vi "COD主界面（列队使用）.vi"() -> (8 "多列列表框":i32(listbox))   [LabVIEW 2016, in "斯坦道CODMn.lvlib"]
uses:
  <vilib>/Utility/miscctls.llb/LVPointTypeDef.ctl
  <vilib>/Plasmionique/MB Master/MB_Master_Serial/MB_Master_Serial.lvclass
  D:/Program Files (x86)/National Instruments/LabVIEW 2016/vi.lib/Plasmionique/MB Master/MB_Master/MB_Master.lvclass
  <vilib>/Plasmionique/MB Master/MB Master.lvlib
  <vilib>/ptbypt/NI_PtbyPt.lvlib
  PLC/PLC.lvlib
panel:
  out "测量数据区":T1 {"单位" items=["ug/L", "mg/L", "ppm", "mg/m3", "cm", "ppb", "ug/m3", "%", "nmol/mol", "umol/mol", "MPN/L", "MPN/100ml", "ng/m3", "NTU", "无量纲", "ms/cm", "us/cm", "℃", "mV", "万个/L"]}
  out "启动选择 3":u16(ring) items=["水样测试", "标样核查", "零点核查", "加标回收", "平行样", "校零", "校标", ""]
  out "加热":bool
  out "搅拌":bool
  out "进硫酸":bool
  out "进草酸钠":bool
  out "进高锰酸钾":bool
  out "进加标回收样":bool
  out "进质控样":bool
  out "进标液":bool
  out "进蒸馏水":bool
  out "进水样":bool
  in  "定时启动":bool
  out "设置值":dbl
  out "系统时间":timestamp
  in  "时间校准":bool
  out "仪器时间":timestamp
  in  "修正系数 2":dbl
  in  "浓度 2":dbl
  in  "温度":dbl
  out "秒":u16
  out "分":u16
  in  "data in":T2
  out "数值":i32
  out "报警簇":T3
  out "读取参数":u16[](array[numeric])
  out "循环次数":i32
  out "DATABASE":u16[](array[numeric])
  out "Registers":u16[](array[numeric])
  in  "枚举":enum16{"读取数据", "写入数据", "读取写入DATABASE", "读取参数"}(ring)
  in  "Slave ID":u8=1
  in  "Serial Config":T4={"baud rate (bps)"=115200, "stop bits"=10, "parity"=0, "flow control"=0, "timeout"=1000, "retries"=1} {"stop bits" items=["1.0"=10, "1.5"=15, "2.0"=20]; "flow control" items=["None", "XON/XOFF", "RTS/CTS", "XON/XOFF & RTS/CTS", "DTR/DSR", "XON/XOFF & DTR/DSR"]; "parity" items=["None", "Odd", "Even", "Mark", "Space"]}
  out "COD浓度（mg/L)":dbl
  out "table 输入":string
  out "columns":string[](array[string])
  in  "保存":bool
  out "data":T5
  in  "温度 2":dbl
  in  "恒温时间":dbl
  in  "浓度":dbl
  in  "修正系数":dbl
  in  "基本量程":enum16{"10mL", "20mL"}(ring)
  in  "水样":dbl
  in  "蒸馏水":dbl
  in  "标液":dbl
  in  "质控样":dbl
  in  "加标回收":dbl
  in  "草酸钠":dbl
  in  "高锰酸钾":dbl
  in  "硫酸":dbl
  in  "关闭":bool
  in  "零点泵计量数 2":dbl
  in  "标度泵计量数 2":dbl
  in  "标样浓度 2":dbl
  out "进样管":dbl
  out "高锰酸钾":dbl
  out "草酸钠":dbl
  out "硫酸":dbl
  out "标度滴定值":dbl
  out "零点滴定值":dbl
  in  "启动":bool
  in  "故障清除":bool
  out "排液故障":bool
  out "进水样超量程":bool
  out "模式（受控）":u16
  out "ORP显示":dbl
  out "温度":dbl
  out "标样核查标记":bool
  out "平行样测量":bool
  out "加标回收测量":bool
  out "质控样测量":bool
  out "待机":bool
  out "校标错误":bool
  out "校零错误":bool
  out "测量错误":bool
  out "草酸钠报警":bool
  out "高锰酸钾报警":bool
  out "加热故障":bool
  out "温控器故障":bool
  out "ORP故障":bool
  out "排液标记":bool
  out "故障标记":bool
  out "校标标记":bool
  out "校零标记":bool
  out "通讯状态":bool
  out "水样测量":bool
  in  "参数配置":bool
  in  "VISA resource name":refnum<visa-resource-name>="COM4" caption="VISA资源名称"
  in  "停止":bool
  in  "单步启动":bool
  # "测量时间："
  # "水样~加标回收"
  # "mV"
  # "℃"
  # "注：遇到加热故障和排液故障时仪器不能正常启动，\n必须排查故障并点击报警清除按钮方可运行。"
  # "基本参数设置"
  # "泵计量参数设置"
  # "校零校标结果"
  # "加热恒温温度（℃）："
  # "水样："
  # "高锰酸钾："
  # "校零结果："
  # "校零滴定值："
  # "恒温时间（分钟）："
  # "蒸馏水："
  # "草酸钠："
  # "校标结果："
  # "标度滴定值："
  # "零点泵计量值："
  # "标准液浓度（mg/L）："
  # "标液："
  # "硫酸："
  # "标样浓度："
  # "标度泵计量值："
  # "修正系数："
  # "质控样："
  # "加标回收样："
  # "基本量程（20mL可选）："
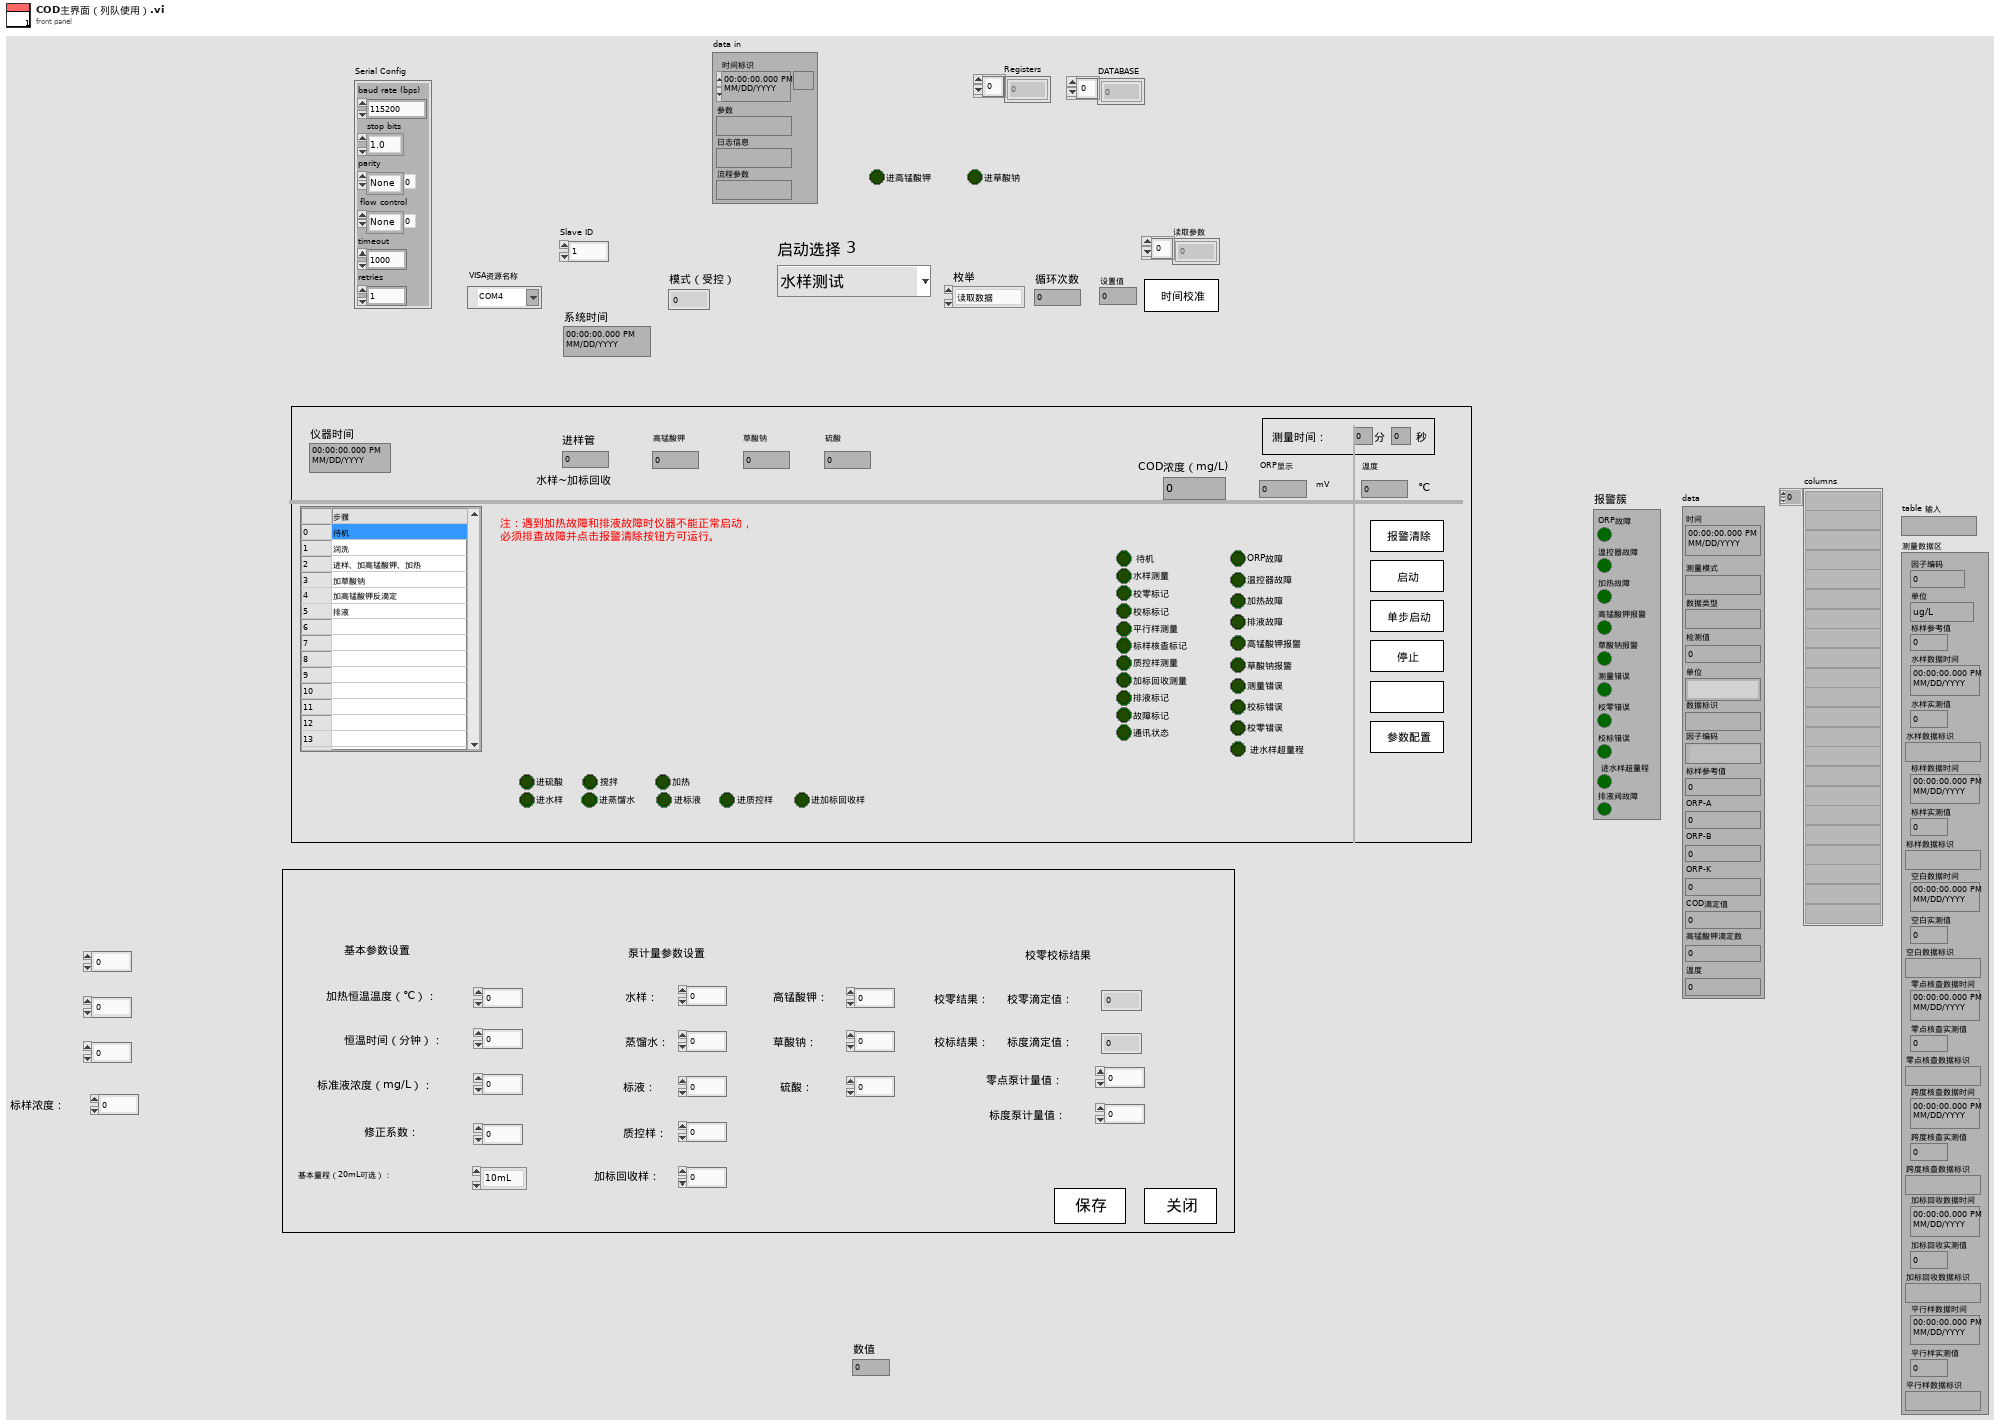
[diagram p1: front panel]
types:
  T1 = cluster{"因子编码":u32, "单位":u16, "标样参考值":sgl, "水样数据时间":timestamp, "水样实测值":sgl, "水样数据标识":string, "标样数据时间":timestamp, "标样实测值":sgl, "标样数据标识":string, "空白数据时间":timestamp, "空白实测值":sgl, "空白数据标识":string, "零点核查数据时间":timestamp, "零点核查实测值":sgl, "零点核查数据标识":string, "跨度核查数据时间":timestamp, "跨度核查实测值":sgl, "跨度核查数据标识":string, "加标回收数据时间":timestamp, "加标回收实测值":sgl, "加标回收数据标识":string, "平行样数据时间":timestamp, "平行样实测值":sgl, "平行样数据标识":string}
  T2 = cluster{"时间标识":timestamp, "参数":string, "日志信息":string, "流程参数":string}
  T3 = cluster{"ORP故障":bool, "温控器故障":bool, "加热故障":bool, "高锰酸钾报警":bool, "草酸钠报警":bool, "测量错误":bool, "校零错误":bool, "校标错误":bool, " 进水样超量程":bool, "排液阀故障":bool}
  T4 = cluster{"baud rate (bps)":u32, "stop bits":u16, "parity":u16, "flow control":u16, "timeout":u32, "retries":i32}
  T5 = cluster{"时间":timestamp, "测量模式":string, "数据类型":string, "检测值":sgl, "单位":string, "数据标识":string, "因子编码":string, "标样参考值":sgl, "ORP-A":sgl, "ORP-B":sgl, "ORP-K":sgl, "COD滴定值":sgl, "高锰酸钾滴定数":sgl, "温度":sgl}
  T6 = cluster{"starting address":u16, "number of holding registers":u16}
  T7 = typedef "LVPointTypeDef.ctl" = cluster{"Horizontal":i16, "Vertical":i16}
  T8 = cluster{"测量模式":enum16{"水样测量", "标样核查", "零点核查", "加标回收", "平行样", "校零", "校标"}}
  T9 = cluster{"时间标识":timestamp, "设备":string, "日志信息":string}
  T10 = cluster{"时间标识":timestamp, "设备":string, "日志信息":string, "流程参数":string}
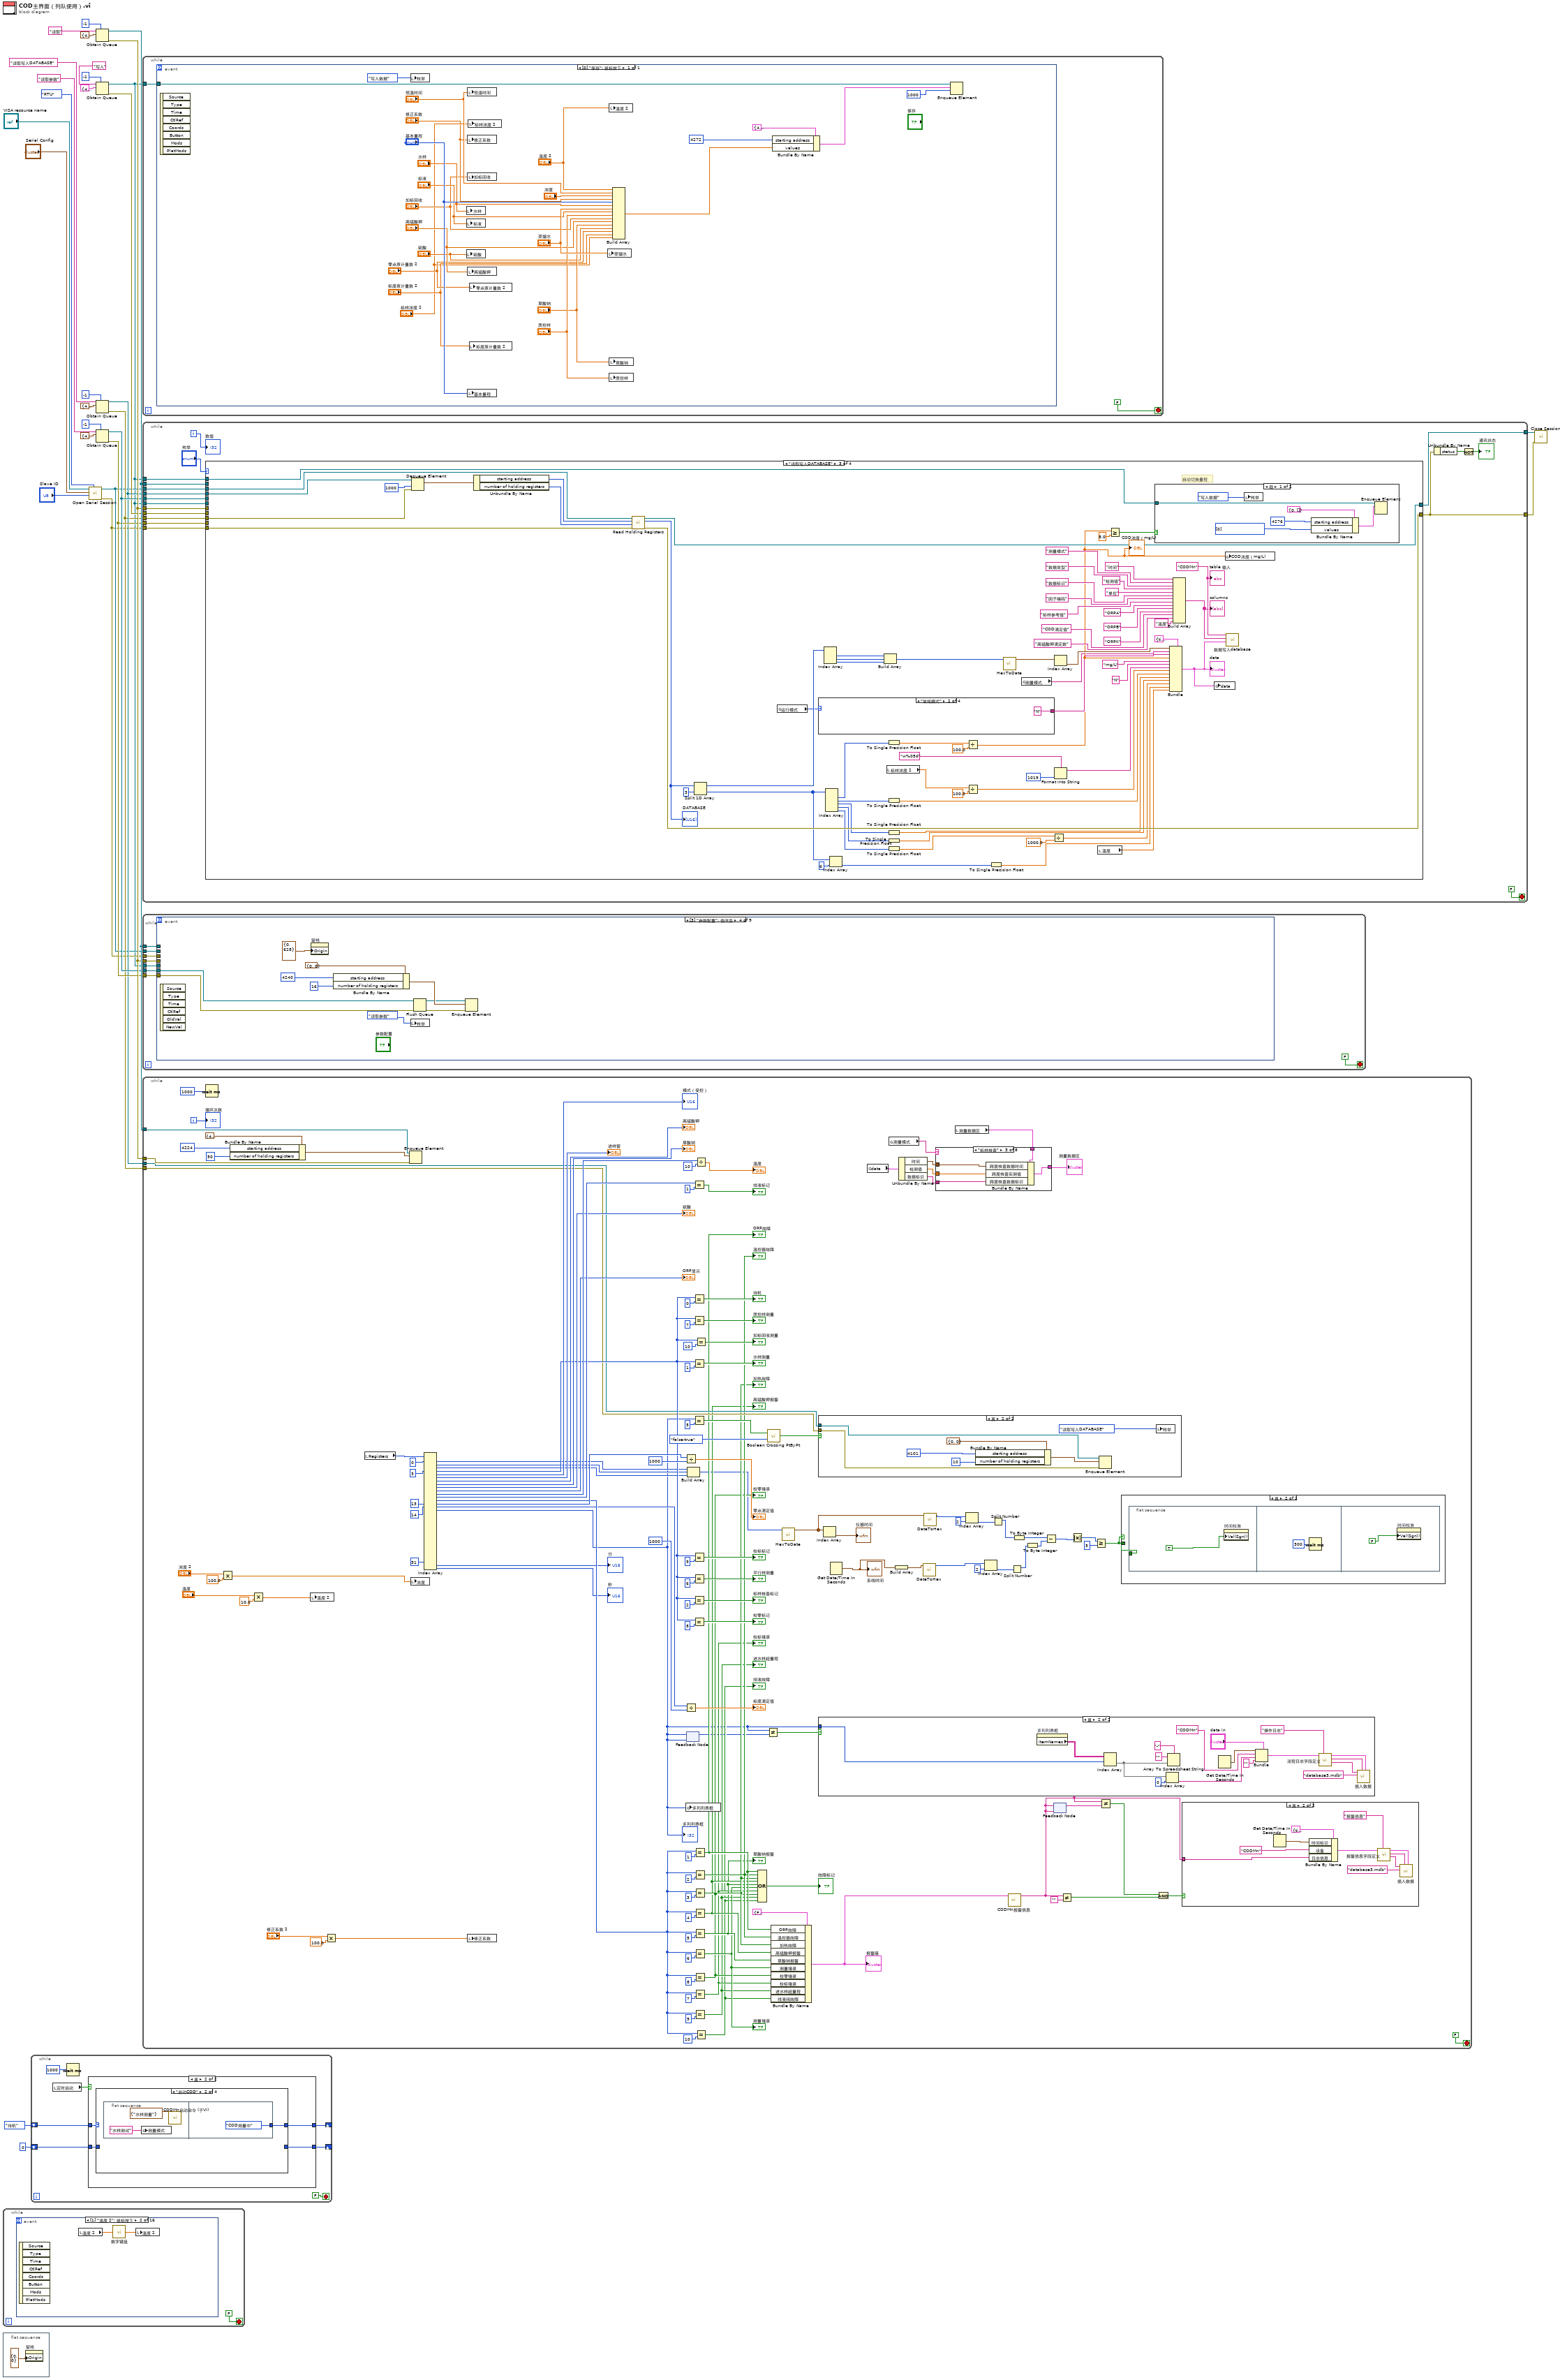
[diagram p0: block diagram]
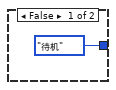
[diagram p2: hidden frame]
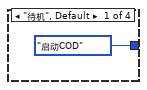
[diagram p3: hidden frame]
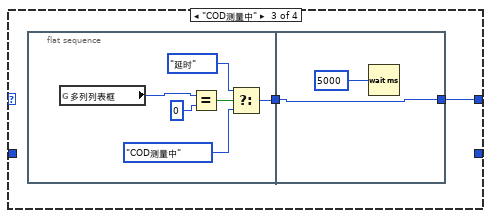
[diagram p4: hidden frame]
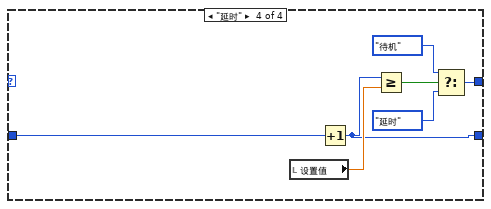
[diagram p5: hidden frame]
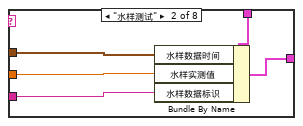
[diagram p7: hidden frame]
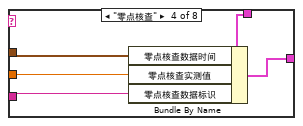
[diagram p8: hidden frame]
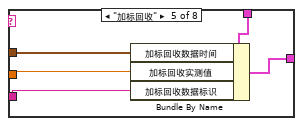
[diagram p9: hidden frame]
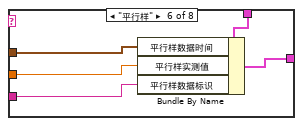
[diagram p10: hidden frame]
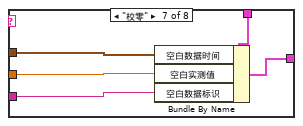
[diagram p11: hidden frame]
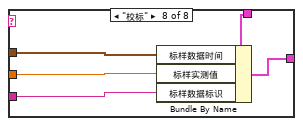
[diagram p12: hidden frame]
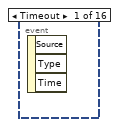
[diagram p17: hidden frame]
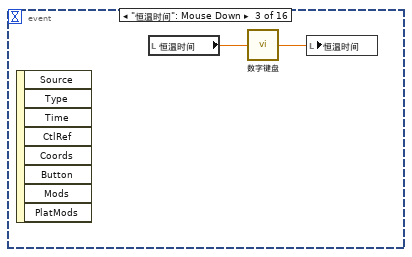
[diagram p18: hidden frame]
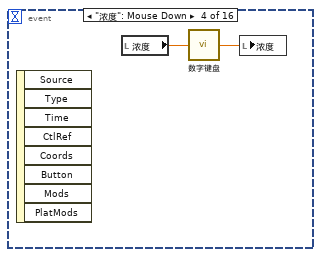
[diagram p19: hidden frame]
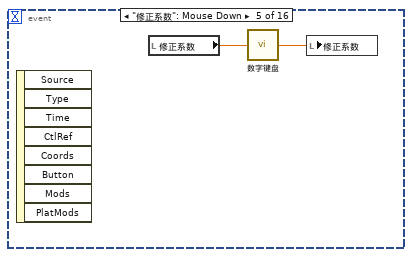
[diagram p20: hidden frame]
diagram:
  n1 = while {
    stop <- FALSE stop-if-true
    n2 = event shown="[1] \"温度 2\": 鼠标按下" {
      selector: _ -> [_ _ _ _ _ _ _ _ _ _ _ _ _ _ _ _]
      dyn-events: _ -> [_ _ _ _ _ _ _ _ _ _ _ _ _ _ _ _]
      timeout: _ -> [_ _ _ _ _ _ _ _ _ _ _ _ _ _ _ _]
      event Timeout {
        n3 = event-data() -> ()  [unwired: 1 in, 3 out]
      }
      event "温度 2": Mouse Down {
        n4 = event-data() -> ()  [unwired: 1 in, 8 out]
        n5 = local read "温度 2"() -> (w32:dbl)
        n6 = call "数字键盘.vi"("OldNumber"=w32) -> ("NewNumber"=w33:sgl)
        n7 = local write "温度 2"(w33) -> ()
      }
      event "恒温时间": Mouse Down {
        n8 = event-data() -> ()  [unwired: 1 in, 8 out]
        n9 = local read "恒温时间"() -> (w34:dbl)
        n10 = call "数字键盘.vi"("OldNumber"=w34) -> ("NewNumber"=w35:sgl)
        n11 = local write "恒温时间"(w35) -> ()
      }
      event "浓度": Mouse Down {
        n12 = event-data() -> ()  [unwired: 1 in, 8 out]
        n13 = local read "浓度"() -> (w36:dbl)
        n14 = call "数字键盘.vi"("OldNumber"=w36) -> ("NewNumber"=w37:sgl)
        n15 = local write "浓度"(w37) -> ()
      }
      event "修正系数": Mouse Down {
        n16 = event-data() -> ()  [unwired: 1 in, 8 out]
        n17 = local read "修正系数"() -> (w38:dbl)
        n18 = call "数字键盘.vi"("OldNumber"=w38) -> ("NewNumber"=w39:sgl)
        n19 = local write "修正系数"(w39) -> ()
      }
      event "水样": Mouse Down {
        n20 = event-data() -> ()  [unwired: 1 in, 8 out]
        n21 = local read "水样"() -> (w40:dbl)
        n22 = call "数字键盘.vi"("OldNumber"=w40) -> ("NewNumber"=w41:sgl)
        n23 = local write "水样"(w41) -> ()
      }
      event "蒸馏水": Mouse Down {
        n24 = event-data() -> ()  [unwired: 1 in, 8 out]
        n25 = local read "蒸馏水"() -> (w42:dbl)
        n26 = call "数字键盘.vi"("OldNumber"=w42) -> ("NewNumber"=w43:sgl)
        n27 = local write "蒸馏水"(w43) -> ()
      }
      event "标液": Mouse Down {
        n28 = event-data() -> ()  [unwired: 1 in, 8 out]
        n29 = local read "标液"() -> (w44:dbl)
        n30 = call "数字键盘.vi"("OldNumber"=w44) -> ("NewNumber"=w45:sgl)
        n31 = local write "标液"(w45) -> ()
      }
      event "质控样": Mouse Down {
        n32 = event-data() -> ()  [unwired: 1 in, 8 out]
        n33 = local read "质控样"() -> (w46:dbl)
        n34 = call "数字键盘.vi"("OldNumber"=w46) -> ("NewNumber"=w47:sgl)
        n35 = local write "质控样"(w47) -> ()
      }
      event "加标回收": Mouse Down {
        n36 = event-data() -> ()  [unwired: 1 in, 8 out]
        n37 = local read "加标回收"() -> (w48:dbl)
        n38 = call "数字键盘.vi"("OldNumber"=w48) -> ("NewNumber"=w49:sgl)
        n39 = local write "加标回收"(w49) -> ()
      }
      event "草酸钠": Mouse Down {
        n40 = event-data() -> ()  [unwired: 1 in, 8 out]
        n41 = local read "草酸钠"() -> (w50:dbl)
        n42 = call "数字键盘.vi"("OldNumber"=w50) -> ("NewNumber"=w51:sgl)
        n43 = local write "草酸钠"(w51) -> ()
      }
      event "高锰酸钾": Mouse Down {
        n44 = event-data() -> ()  [unwired: 1 in, 8 out]
        n45 = local read "高锰酸钾"() -> (w52:dbl)
        n46 = call "数字键盘.vi"("OldNumber"=w52) -> ("NewNumber"=w53:sgl)
        n47 = local write "高锰酸钾"(w53) -> ()
      }
      event "硫酸": Mouse Down {
        n48 = event-data() -> ()  [unwired: 1 in, 8 out]
        n49 = local read "硫酸"() -> (w54:dbl)
        n50 = call "数字键盘.vi"("OldNumber"=w54) -> ("NewNumber"=w55:sgl)
        n51 = local write "硫酸"(w55) -> ()
      }
      event "零点泵计量数 2": Mouse Down {
        n52 = event-data() -> ()  [unwired: 1 in, 8 out]
        n53 = local read "零点泵计量数 2"() -> (w56:dbl)
        n54 = call "数字键盘.vi"("OldNumber"=w56) -> ("NewNumber"=w57:sgl)
        n55 = local write "零点泵计量数 2"(w57) -> ()
      }
      event "标度泵计量数 2": Mouse Down {
        n56 = event-data() -> ()  [unwired: 1 in, 8 out]
        n57 = local read "标度泵计量数 2"() -> (w58:dbl)
        n58 = call "数字键盘.vi"("OldNumber"=w58) -> ("NewNumber"=w59:sgl)
        n59 = local write "标度泵计量数 2"(w59) -> ()
      }
      event "标样浓度 2": Mouse Down {
        n60 = event-data() -> ()  [unwired: 1 in, 8 out]
        n61 = local read "标样浓度 2"() -> (w60:dbl)
        n62 = call "数字键盘.vi"("OldNumber"=w60) -> ("NewNumber"=w61:sgl)
        n63 = local write "标样浓度 2"(w61) -> ()
      }
    }
  }
  n64 = flat-sequence {
    frame #0 {
      n65 = property on="窗格" class="Pane"("Origin"=T7 {"Horizontal"=0, "Vertical"=0} ("原点")) -> ()  [unwired: 2 in, 2 out]
    }
  }
  n66 = while {
    shift-right: [w64] -> _
    shift-left: enum16{"待机", "启动COD", "COD测量中", "延时"}."待机" -> [w66]
    shift-right: [w63] -> _
    shift-left: 0 -> [w65]
    stop <- FALSE stop-if-true
    n67 = local read "定时启动"() -> (w68:bool)
    n68 = Wait (ms)(milliseconds to wait=u32 1000 ("等待时间（毫秒）")) -> ()  [unwired: 1 out]
    n69 = case shown="真" w68 {
      tunnel: w66 -> [_ w74]
      tunnel: w65 -> [_ w73]
      tunnel: [enum16{"待机", "启动COD", "COD测量中", "延时"}."待机" w72] -> w64
      tunnel: [_ w71] -> w63
      frame False {
      }
      frame True {
        n70 = case shown="\"启动COD\"" w74 {
          tunnel: w73 -> [_ _ _ w96]
          tunnel: [enum16{"待机", "启动COD", "COD测量中", "延时"}."启动COD" w76 w81 w90] -> w72
          tunnel: [_ _ _ w93] -> w71
          frame "待机", Default {
          }
          frame "启动COD" {
            n71 = flat-sequence {
              tunnel: [enum16{"待机", "启动COD", "COD测量中", "延时"}."COD测量中"] -> w76
              frame #0 {
                n72 = global write "COD测量模式全局.vi" "测量模式"("水样测试" ("测量模式")) -> ()
                n73 = call "CODMn启动命令 (子VI).vi"("启动测量模式"=T8 {"测量模式"=enum."水样测量"}) -> ()  [unwired: 11 in]
              }
              frame #1 {
              }
            }
          }
          frame "COD测量中" {
            n74 = flat-sequence {
              tunnel: [w82] -> w80
              tunnel: [w89] -> w81
              tunnel: w80 -> [w89]
              frame #0 {
                n75 = global read "运行时序全局变量.vi" "多列列表框"() -> (w87:i32)
                n76 = Equal?(x=w87, y=0) -> (x = y?=w85:bool)
                n77 = Select(t=enum16{"待机", "启动COD", "COD测量中", "延时"}."延时", s=w85, f=enum16{"待机", "启动COD", "COD测量中", "延时"}."COD测量中") -> (s? t:f=w82:enum16{"待机", "启动COD", "COD测量中", "延时"})
              }
              frame #1 {
                n78 = Wait (ms)(milliseconds to wait=u32 5000 ("等待时间（毫秒）")) -> ()  [unwired: 1 out]
              }
            }
          }
          frame "延时" {
            n79 = local read "设置值"() -> (w95:dbl)
            n80 = Increment(x=w96) -> (x+1=w93:i32)
            n81 = Greater Or Equal?(x=w93, y=w95) -> (x >= y?=w94:bool)
            n82 = Select(t=enum16{"待机", "启动COD", "COD测量中", "延时"}."待机", s=w94, f=enum16{"待机", "启动COD", "COD测量中", "延时"}."延时") -> (s? t:f=w90:enum16{"待机", "启动COD", "COD测量中", "延时"})
          }
        }
      }
    }
  }
  n83 = call <vilib>:"Open Serial Session.vi"("Mode (RTU)"=enum16{"RTU", "ASCII"}."RTU", "Slave ID"="Slave ID", "Serial Config"="Serial Config", "VISA Resource"="VISA resource name") -> ("Error out"=w4:errorcluster, "MB_Serial session"=w5:refnum<class "MB_Master_Serial.lvclass">)  [unwired: 6 in]
  n84 = Obtain Queue(max queue size (-1, unlimited)=-1 ("队列最大值（-1，无限）"), name (unnamed)="读取" ("名称（未命名）"), element data type=T6 {"starting address"=4224, "number of holding registers"=16}) -> (queue out=w20:refnum<queue>, error out=w19:errorcluster)  [unwired: 2 in, 1 out]
  n85 = Obtain Queue(max queue size (-1, unlimited)=-1 ("队列最大值（-1，无限）"), name (unnamed)="写入" ("名称（未命名）"), element data type=cluster{"starting address":u16, "values":u16[]} {"starting address"=4272, "values"=[]}) -> (queue out=w1:refnum<queue>, error out=w6:errorcluster)  [unwired: 2 in, 1 out]
  n86 = Obtain Queue(max queue size (-1, unlimited)=-1 ("队列最大值（-1，无限）"), name (unnamed)="读取写入DATABASE" ("名称（未命名）"), element data type=T6 {"starting address"=4224, "number of holding registers"=16}) -> (queue out=w8:refnum<queue>, error out=w7:errorcluster)  [unwired: 2 in, 1 out]
  n87 = Obtain Queue(max queue size (-1, unlimited)=-1 ("队列最大值（-1，无限）"), name (unnamed)="读取参数" ("名称（未命名）"), element data type=T6 {"starting address"=4224, "number of holding registers"=16}) -> (queue out=w13:refnum<queue>, error out=w12:errorcluster)  [unwired: 2 in, 1 out]
  n88 = while {
    tunnel: w1 -> [w98]
    stop <- FALSE stop-if-true
    n89 = event shown="[0] \"保存\": 鼠标按下" {
      selector: _ -> [_]
      dyn-events: _ -> [_]
      timeout: _ -> [_]
      tunnel: w98 -> [w108]
      event "保存": Mouse Down {
        n90 = event-data() -> ()  [unwired: 1 in, 8 out]
        n91 = local write "枚举"(enum16{"读取数据", "写入数据", "读取写入DATABASE", "读取参数"}."写入数据" ("枚举")) -> ()
        n92 = local write "水样"("水样") -> ()
        n93 = local write "标液"("标液") -> ()
        n94 = local write "硫酸"("硫酸") -> ()
        n95 = local write "恒温时间"("恒温时间") -> ()
        n96 = local write "修正系数"("修正系数") -> ()
        n97 = local write "加标回收"("加标回收") -> ()
        n98 = local write "高锰酸钾"("高锰酸钾") -> ()
        n99 = local write "基本量程"("基本量程") -> ()
        n100 = local write "标样浓度 2"("标样浓度 2") -> ()
        n101 = local write "零点泵计量数 2"("零点泵计量数 2") -> ()
        n102 = local write "标度泵计量数 2"("标度泵计量数 2") -> ()
        n103 = local write "蒸馏水"("蒸馏水") -> ()
        n104 = local write "温度 2"("温度 2") -> ()
        n105 = local write "草酸钠"("草酸钠") -> ()
        n106 = local write "质控样"("质控样") -> ()
        n107 = Build Array("温度 2", "恒温时间", "浓度", "修正系数", "基本量程", "水样", "蒸馏水", "标液", "质控样", "加标回收", "高锰酸钾", "草酸钠", "硫酸", "零点泵计量数 2", "标度泵计量数 2", "标样浓度 2") -> (w106:dbl[])
        n108 = Bundle By Name(cluster=cluster{"starting address":u16, "values":u16[]} {"starting address"=4272, "values"=[]}, "starting address"=u16 4272, "values"=w106) -> (w104:cluster{"starting address":u16, "values":u16[]})
        n109 = Enqueue Element(queue=w108, element=w104, timeout in ms (-1)=1000 ("超时毫秒(-1)")) -> ()  [unwired: 1 in, 3 out]
      }
    }
  }
  n110 = while {
    tunnel: w5 -> [w139]
    tunnel: w4 -> [w138]
    tunnel: w1 -> [w137]
    tunnel: w20 -> [w136]
    tunnel: w19 -> [w135]
    tunnel: [w125] -> w18
    tunnel: [w134] -> w17
    tunnel: w13 -> [w132]
    tunnel: w12 -> [w131]
    tunnel: w8 -> [w130]
    tunnel: w7 -> [w129]
    tunnel: w6 -> [w128]
    tunnel: w1 -> [w122]
    i -> [w124]
    stop <- FALSE stop-if-true
    n111 = case shown="\"读取写入DATABASE\"" "枚举" {
      tunnel: w139 -> [w175 w183 w261 w310]
      tunnel: w138 -> [w174 w179 w260 w309]
      tunnel: w137 -> [_ w182 _ _]
      tunnel: [w148 w181 w263 w312] -> w134
      tunnel: [w147 w180 w262 w311] -> w125
      tunnel: w136 -> [w172 _ _ _]
      tunnel: w135 -> [w168 _ _ _]
      tunnel: w132 -> [_ _ _ w308]
      tunnel: w131 -> [_ _ _ w307]
      tunnel: w130 -> [_ _ w259 _]
      tunnel: w129 -> [_ _ w258 _]
      tunnel: w128 -> [_ w178 _ _]
      tunnel: w122 -> [_ _ w200 _]
      frame "读取数据", Default {
        n112 = Dequeue Element(queue=w172, timeout in ms (-1)=1000 ("超时毫秒(-1)"), error in (no error)=w168) -> (element=w171:T6)  [unwired: 3 out]
        n113 = Unbundle By Name(w171) -> ("starting address"=w170:u16, "number of holding registers"=w169:u16)
        n114 = call <vilib>:"Read Holding Registers.vi"("error in (no error)"=w174, "quantity"=w169, "starting address"=w170, "MB session in"=w175) -> ("error out"=w163:errorcluster, "Registers"=→"Registers":u16[], "MB session out"=w166:refnum<class "MB_Master_Serial.lvclass">)  [unwired: 5 in]
        n115 = call <vilib>:"Read Coils.vi"("error in (no error)"=w163, "quantity"=u16 8, "starting address"=u16 140, "MB session in"=w166) -> ("error out"=w153:errorcluster, "Coils"=w162:bool[], "MB session out"=w154:refnum<class "MB_Master_Serial.lvclass">)  [unwired: 5 in]
        n116 = Index Array(array=w162) -> (element #1=→"进水样":bool, element #2=→"进蒸馏水":bool, element #3=→"进标液":bool, element #4=→"进质控样":bool, element #5=→"进加标回收样":bool, element #6=→"进高锰酸钾":bool, element #7=→"进草酸钠":bool, element #8=→"进硫酸":bool)  [unwired: 9 in, 1 out]
        n117 = call <vilib>:"Read Coils.vi"("error in (no error)"=w153, "quantity"=u16 1, "starting address"=u16 137, "MB session in"=w154) -> ("error out"=w149:errorcluster, "Coils"=w141:bool[], "MB session out"=w150:refnum<class "MB_Master_Serial.lvclass">)  [unwired: 5 in]
        n118 = Index Array(array=w141) -> (element=→"搅拌":bool)  [unwired: 1 in]
        n119 = call <vilib>:"Read Coils.vi"("error in (no error)"=w149, "quantity"=u16 1, "starting address"=u16 400, "MB session in"=w150) -> ("error out"=w147:errorcluster, "Coils"=w144:bool[], "MB session out"=w148:refnum<class "MB_Master_Serial.lvclass">)  [unwired: 5 in]
        n120 = Index Array(array=w144) -> (element=→"加热":bool)  [unwired: 1 in]
      }
      frame "写入数据" {
        n121 = flat-sequence {
          tunnel: w183 -> [w193]
          tunnel: w182 -> [w192]
          tunnel: w179 -> [w186]
          tunnel: w178 -> [w185]
          tunnel: [w188] -> w177
          tunnel: [w187] -> w176
          tunnel: [w195] -> w180
          tunnel: [w196] -> w181
          tunnel: w177 -> [w196]
          tunnel: w176 -> [w195]
          frame #0 {
            n122 = Dequeue Element(queue=w192, error in (no error)=w185) -> (queue out=w184:refnum<queue>, element=w191:cluster{"starting address":u16, "values":u16[]})  [unwired: 1 in, 2 out]
            n123 = Flush Queue(queue=w184) -> ()  [unwired: 1 in, 3 out]
            n124 = Unbundle By Name(w191) -> ("starting address"=w190:u16, "values"=w189:u16[])
            n125 = call <vilib>:"Write Multiple Registers.vi"("error in (no error)"=w186, "values"=w189, "starting address"=w190, "MB session in"=w193) -> ("error out"=w187:errorcluster, "MB session out"=w188:refnum<class "MB_Master_Serial.lvclass">)  [unwired: 6 in]
          }
          frame #1 {
            n126 = local write "枚举"(enum16{"读取数据", "写入数据", "读取写入DATABASE", "读取参数"}."读取数据" ("枚举")) -> ()
          }
        }
      }
      frame "读取写入DATABASE" {
        w226 = "CODMn" ("table")
        # "自动切换量程"
        n127 = Dequeue Element(queue=w259, timeout in ms (-1)=1000 ("超时毫秒(-1)"), error in (no error)=w258) -> (element=w266:T6)  [unwired: 3 out]
        n128 = Unbundle By Name(w266) -> ("starting address"=w265:u16, "number of holding registers"=w264:u16)
        n129 = call <vilib>:"Read Holding Registers.vi"("error in (no error)"=w260, "quantity"=w264, "starting address"=w265, "MB session in"=w261) -> ("error out"=w262:errorcluster, "Registers"=w222:u16[], "MB session out"=w263:refnum<class "MB_Master_Serial.lvclass">)  [unwired: 5 in]
        "DATABASE" <- w222
        n130 = Split 1D Array(array=w222, index=3 ("索引")) -> (first subarray=w256:u16[], second subarray=w244:u16[])
        n131 = global read "系统变量.vi" "运行模式"() -> (w205:enum16{"维护模式", "常规模式", "应急模式", "质控模式"})
        n132 = case shown="\"常规模式\"" w205 {
          tunnel: ["M" ("单位") "N" ("单位") "hd" ("单位") "hd" ("单位")] -> w204
          frame "维护模式", Default {
          }
          frame "常规模式" {
          }
          frame "应急模式" {
          }
          frame "质控模式" {
          }
        }
        n133 = Index Array(array=w256) -> (element #1=w254:u16, element #2=w253:u16, element #3=w252:u16)  [unwired: 3 in]
        n134 = Index Array(array=w244) -> (element #1=w249:u16, element #2=w248:u16, element #3=w247:u16, element #4=w246:u16, element #5=w245:u16)  [unwired: 5 in]
        n135 = Index Array(array=w244, index=6 ("索引")) -> (element=w242:u16)
        n136 = Build Array(w254, w253, w252) -> (w251:u16[])
        n137 = local read "标样浓度 2"() -> (w220:dbl)
        n138 = To Single Precision Float(number=w249) -> (single precision float=w241:sgl)
        n139 = To Single Precision Float(number=w248) -> (single precision float=w210:sgl)
        n140 = To Single Precision Float(number=w247) -> (single precision float=w211:sgl)
        n141 = To Single Precision Float(number=w246) -> (single precision float=w212:sgl)
        n142 = To Single Precision Float(number=w245) -> (single precision float=w238:sgl)
        n143 = Divide(x=w241, y=sgl 100.0) -> (x/y=w198:sgl)
        "COD浓度（mg/L)" <- w198
        n144 = Divide(x=w220, y=100.0) -> (x/y=w209:dbl)
        n145 = To Single Precision Float(number=w242) -> (single precision float=w214:sgl)
        n146 = call "HexToDate.vi"("数组"=w251) -> ("DATE"=w255:timestamp[])  [unwired: 10 in]
        n147 = global read "COD测量模式全局.vi" "测量模式"() -> (w197:string)
        n148 = Divide(x=w238, y=sgl 1000.0) -> (x/y=w213:sgl)
        n149 = Index Array(array=w255) -> (element=w250:timestamp)  [unwired: 1 in]
        n150 = Format Into String(format string="w%05d" ("格式字符串"), u32 1019 ("因子编码")) -> (resulting string=w208:string)  [unwired: 2 in, 1 out]
        n151 = local read "温度"() -> (w203:dbl)
        n152 = Greater Or Equal?(x=w198, y=sgl 8.0) -> (x >= y?=w201:bool)
        n153 = case shown="假" w201 {
          tunnel: w200 -> [w267 w276]
          frame False {
            n154 = local write "枚举"(enum16{"读取数据", "写入数据", "读取写入DATABASE", "读取参数"}."写入数据" ("枚举")) -> ()
            n155 = Bundle By Name(cluster=cluster{"starting address":u16, "values":u16[]} {"starting address"=0, "values"=[]}, "starting address"=u16 4276, "values"=u16[] [0]) -> (w270:cluster{"starting address":u16, "values":u16[]})
            n156 = Enqueue Element(queue=w267, element=w270) -> ()  [unwired: 2 in, 3 out]
          }
          frame True {
            n157 = local write "枚举"(enum16{"读取数据", "写入数据", "读取写入DATABASE", "读取参数"}."写入数据" ("枚举")) -> ()
            n158 = Bundle By Name(cluster=cluster{"starting address":u16, "values":u16[]} {"starting address"=0, "values"=[]}, "starting address"=u16 4276, "values"=u16[] [1]) -> (w277:cluster{"starting address":u16, "values":u16[]})
            n159 = Enqueue Element(queue=w276, element=w277) -> ()  [unwired: 2 in, 3 out]
          }
        }
        n160 = Bundle(cluster=T5 {"时间"=timestamp(0 s since 1904-01-01), "测量模式"="", "数据类型"="", "检测值"=0.0, "单位"="", "数据标识"="", "因子编码"="", "标样参考值"=0.0, "ORP-A"=0.0, "ORP-B"=0.0, "ORP-K"=0.0, "COD滴定值"=0.0, "高锰酸钾滴定数"=0.0, "温度"=0.0} ("data"), "时间"=w250, "测量模式"=w197, "数据类型"=w204, "检测值"=w198, "单位"="mg/L", "数据标识"="N", "因子编码"=w208, "标样参考值"=w209, "ORP-A"=w210, "ORP-B"=w211, "ORP-K"=w212, "COD滴定值"=w213, "高锰酸钾滴定数"=w214, "温度"=w203) -> (w199:T5)
        "data" <- w199
        n161 = Build Array("时间", "测量模式", "数据类型", "检测值", "单位", "数据标识", "因子编码", "标样参考值", "ORPA", "ORPB", "ORPK", "COD滴定值", "高锰酸钾滴定数", "温度") -> (w225:string[])
        "columns" <- w225
        n162 = global write "COD读取DATA全局.vi" "data"(w199) -> ()
        n163 = global write "COD浓度全局变量.vi" "COD浓度（mg/L)"(w198) -> ()
        n164 = call "数据写入database.vi"("data"=w199, "columns"=w225, "table"=w226) -> ()  [unwired: 9 in]
        "table 输入" <- w226
      }
      frame "读取参数" {
        n165 = Dequeue Element(queue=w308, timeout in ms (-1)=1000 ("超时毫秒(-1)"), error in (no error)=w307) -> (element=w316:T6)  [unwired: 3 out]
        n166 = local write "枚举"(enum16{"读取数据", "写入数据", "读取写入DATABASE", "读取参数"}."读取数据" ("枚举")) -> ()
        n167 = Unbundle By Name(w316) -> ("starting address"=w315:u16, "number of holding registers"=w314:u16)
        n168 = call <vilib>:"Read Holding Registers.vi"("error in (no error)"=w309, "quantity"=w314, "starting address"=w315, "MB session in"=w310) -> ("error out"=w311:errorcluster, "Registers"=w293:u16[], "MB session out"=w312:refnum<class "MB_Master_Serial.lvclass">)  [unwired: 5 in]
        "读取参数" <- w293
        n169 = Index Array(array=w293) -> (element #1=w286:u16, element #2=w306:u16, element #3=w305:u16, element #4=w284:u16, element #5=w304:u16, element #6=w303:u16, element #7=w302:u16, element #8=w301:u16, element #9=w300:u16, element #10=w299:u16, element #11=w298:u16, element #12=w297:u16, element #13=w296:u16, element #14=w295:u16, element #15=w294:u16, element #16=w291:u16)  [unwired: 16 in]
        n170 = local write "浓度"(w305) -> ()
        n171 = local write "水样"(w303) -> ()
        n172 = local write "硫酸"(w296) -> ()
        n173 = local write "标液"(w301) -> ()
        n174 = local write "草酸钠"(w297) -> ()
        n175 = local write "蒸馏水"(w302) -> ()
        n176 = local write "质控样"(w300) -> ()
        n177 = local write "恒温时间"(w306) -> ()
        n178 = local write "基本量程"(w304) -> ()
        n179 = local write "加标回收"(w299) -> ()
        n180 = local write "高锰酸钾"(w298) -> ()
        n181 = local write "零点泵计量数 2"(w295) -> ()
        n182 = local write "标度泵计量数 2"(w294) -> ()
        n183 = Divide(x=w286, y=u16 10) -> (x/y=w287:dbl)
        n184 = Divide(x=w284, y=u16 100) -> (x/y=w283:dbl)
        n185 = Divide(x=w291, y=u16 100) -> (x/y=w290:dbl)
        n186 = local write "温度"(w287) -> ()
        n187 = local write "浓度 2"(w290) -> ()
        n188 = local write "修正系数 2"(w283) -> ()
      }
    }
    n189 = Unbundle By Name(w125) -> ("status"=w126:bool)
    n190 = Not(x=w126) -> (.not. x?=→"通讯状态":bool)
    "数值" <- w124
  }
  n191 = while {
    tunnel: w20 -> [w324]
    tunnel: w19 -> [w323]
    tunnel: w1 -> [w322]
    tunnel: w13 -> [w321]
    tunnel: w12 -> [w320]
    tunnel: w5 -> [w318]
    tunnel: w4 -> [w317]
    stop <- FALSE stop-if-true
    n192 = event shown="[3] \"参数配置\": 值改变" {
      selector: _ -> [_ _ _ _ _ _ _ _ _]
      dyn-events: _ -> [_ _ _ _ _ _ _ _ _]
      timeout: _ -> [_ _ _ _ _ _ _ _ _]
      tunnel: w324 -> [_ _ _ _ _ _ _ _ _]
      tunnel: w323 -> [_ _ _ _ _ _ _ _ _]
      tunnel: w322 -> [w331 w365 w388 _ _ _ w406 w420 _]
      tunnel: w321 -> [_ _ _ w394 _ _ _ _ _]
      tunnel: w320 -> [_ _ _ w393 _ _ _ _ _]
      tunnel: w318 -> [_ _ _ _ _ w405 _ _ _]
      tunnel: w317 -> [_ _ _ _ _ w404 _ _ _]
      event "单步启动": Mouse Down {
        n193 = event-data() -> ()  [unwired: 1 in, 8 out]
        n194 = call "单步启动选择对话框.vi"() -> ("启动选择 2"=w334:u16)  [unwired: 10 in, 1 out]
        n195 = case shown="0" w334 {
          tunnel: [u16 4610 ("address") u16 4610 ("address") u16 4610 ("address") u16 4610 ("address") u16 4610 ("address") u16 4610 ("address") u16 4610 ("address") u16 4610 ("address") u16 4610 ("address") u16 4610 ("address") u16 4610 ("address") u16 4610 ("address")] -> w330
          tunnel: [u16 1 ("address") u16 2 ("address") u16 3 ("address") u16 4 ("address") u16 5 ("address") u16 6 ("address") u16 7 ("address") u16 8 ("address") u16 9 ("holding register value") u16 10 ("holding register value") u16 11 ("holding register value") u16 0 ("address")] -> w327
          frame 0 {
          }
          frame 1 {
          }
          frame 2 {
          }
          frame 3 {
          }
          frame 4 {
          }
          frame 5 {
          }
          frame 6 {
          }
          frame 7 {
          }
          frame 8 {
          }
          frame 9 {
          }
          frame 10 {
          }
          frame 11, Default {
          }
        }
        n196 = local write "枚举"(enum16{"读取数据", "写入数据", "读取写入DATABASE", "读取参数"}."写入数据" ("枚举")) -> ()
        n197 = Insert Into Array(array=u16[] [] ("values"), index=0 ("索引"), new element=w327) -> (w326:u16[])
        n198 = Bundle By Name(cluster=cluster{"starting address":u16, "values":u16[]} {"starting address"=0, "values"=[]}, "starting address"=w330, "values"=w326) -> (w332:cluster{"starting address":u16, "values":u16[]})
        n199 = Enqueue Element(queue=w331, element=w332) -> ()  [unwired: 2 in, 3 out]
      }
      event "启动": Mouse Down {
        n200 = event-data() -> ()  [unwired: 1 in, 8 out]
        n201 = flat-sequence {
          tunnel: [w369] -> w368
          frame #0 {
            n202 = call "启动测量模式选择对话框.vi"() -> ("启动选择 3"=w369:u16)  [unwired: 11 in]
            "启动选择 3" <- w369
          }
          frame #1 {
            n203 = property on="启动选择 3" class="Ring (严格)"() -> ("RingText.Text"=w370:string)  [unwired: 2 in, 2 out]
            n204 = global write "COD测量模式全局.vi" "测量模式"(w370) -> ()
          }
        }
        n205 = case shown="7, 默认" w368 {
          tunnel: [u16 4608 ("address") u16 4608 ("address") u16 4608 ("address") u16 4608 ("address") u16 4608 ("address") u16 4608 ("address") u16 4608 ("address") u16 4608 ("address")] -> w364
          tunnel: [u16 1 ("address") u16 2 ("address") u16 3 ("address") u16 7 ("address") u16 6 ("address") u16 8 ("address") u16 9 ("address") u16 0 ("address")] -> w361
          frame 0 {
          }
          frame 1 {
          }
          frame 2 {
          }
          frame 3 {
          }
          frame 4 {
          }
          frame 5 {
          }
          frame 6 {
          }
          frame 7, Default {
          }
        }
        n206 = local write "枚举"(enum16{"读取数据", "写入数据", "读取写入DATABASE", "读取参数"}."写入数据" ("枚举")) -> ()
        n207 = Insert Into Array(array=u16[] [] ("values"), index=0 ("索引"), new element=w361) -> (w360:u16[])
        n208 = Bundle By Name(cluster=cluster{"starting address":u16, "values":u16[]} {"starting address"=0, "values"=[]}, "starting address"=w364, "values"=w360) -> (w366:cluster{"starting address":u16, "values":u16[]})
        n209 = Enqueue Element(queue=w365, element=w366) -> ()  [unwired: 2 in, 3 out]
      }
      event "停止": Value Change {
        n210 = event-data() -> ()  [unwired: 1 in, 6 out]
        n211 = local write "枚举"(enum16{"读取数据", "写入数据", "读取写入DATABASE", "读取参数"}."写入数据" ("枚举")) -> ()
        n212 = Bundle By Name(cluster=cluster{"starting address":u16, "values":u16[]} {"starting address"=0, "values"=[]}, "starting address"=u16 4608, "values"=u16[] [11]) -> (w390:cluster{"starting address":u16, "values":u16[]})
        n213 = Enqueue Element(queue=w388, element=w390) -> ()  [unwired: 2 in, 3 out]
      }
      event "参数配置": Value Change {
        n214 = event-data() -> ()  [unwired: 1 in, 6 out]
        n215 = property on="窗格" class="Pane"("Origin"=T7 {"Horizontal"=0, "Vertical"=628} ("原点")) -> ()  [unwired: 2 in, 2 out]
        n216 = Bundle By Name(cluster=T6 {"starting address"=0, "number of holding registers"=0}, "starting address"=u16 4240, "number of holding registers"=u16 16) -> (w401:T6)
        n217 = local write "枚举"(enum16{"读取数据", "写入数据", "读取写入DATABASE", "读取参数"}."读取参数" ("枚举")) -> ()
        n218 = Flush Queue(queue=w394, error in (no error)=w393) -> (queue out=w397:refnum<queue>, error out=w396:errorcluster)  [unwired: 1 out]
        n219 = Enqueue Element(queue=w397, element=w401, error in (no error)=w396) -> ()  [unwired: 1 in, 3 out]
      }
      event "关闭": Value Change {
        n220 = event-data() -> ()  [unwired: 1 in, 6 out]
        n221 = property on="窗格" class="Pane"("Origin"=T7 {"Horizontal"=0, "Vertical"=0} ("原点")) -> ()  [unwired: 2 in, 2 out]
      }
      event Timeout; Application Instance Close {
        n222 = event-data() -> ()  [unwired: 1 in, 3 out]
        n223 = call-dynamic "Close Session.vi"("error in (no error)"=w404, "MB_Serial session"=w405) -> ()  [unwired: 9 in, 1 out]
      }
      event "时间校准": Value Change {
        n224 = event-data() -> ()  [unwired: 1 in, 6 out]
        n225 = flat-sequence {
          tunnel: w406 -> [w411]
          frame #0 {
            n226 = Get Date/Time In Seconds() -> (seconds since 1Jan1904=w416:timestamp)
            n227 = Build Array(w416) -> (w415:timestamp[])
            n228 = call "DateToHex.vi"("DATE"=w415) -> ("数组"=w409:u16[])  [unwired: 10 in]
            n229 = Insert Into Array(array=u16[] [1] ("values"), index=1 ("索引"), new element=w409) -> (w407:u16[])
            n230 = Bundle By Name(cluster=cluster{"starting address":u16, "values":u16[]} {"starting address"=0, "values"=[]}, "starting address"=u16 4612, "values"=w407) -> (w412:cluster{"starting address":u16, "values":u16[]})
            n231 = Enqueue Element(queue=w411, element=w412) -> ()  [unwired: 2 in, 3 out]
          }
          frame #1 {
            n232 = local write "枚举"(enum16{"读取数据", "写入数据", "读取写入DATABASE", "读取参数"}."写入数据" ("枚举")) -> ()
          }
        }
      }
      event "故障清除": Value Change {
        n233 = event-data() -> ()  [unwired: 1 in, 6 out]
        n234 = local write "枚举"(enum16{"读取数据", "写入数据", "读取写入DATABASE", "读取参数"}."写入数据" ("枚举")) -> ()
        n235 = Bundle By Name(cluster=cluster{"starting address":u16, "values":u16[]} {"starting address"=0, "values"=[]}, "starting address"=u16 4611, "values"=u16[] [1]) -> (w421:cluster{"starting address":u16, "values":u16[]})
        n236 = Enqueue Element(queue=w420, element=w421) -> ()  [unwired: 2 in, 3 out]
      }
      event "定时启动": Mouse Down {
        n237 = event-data() -> ()  [unwired: 1 in, 8 out]
        n238 = call "COD定时启动对话框.vi"() -> ("设置值"=→"设置值":dbl, "确定输出"=w424:bool)  [unwired: 10 in]
        n239 = local write "定时启动"(w424) -> ()
      }
    }
  }
  n240 = while {
    tunnel: w20 -> [w496]
    tunnel: w19 -> [w495]
    tunnel: w8 -> [w490]
    tunnel: w7 -> [w489]
    i -> [w491]
    stop <- FALSE stop-if-true
    n241 = Wait (ms)(milliseconds to wait=u32 1000 ("等待时间（毫秒）")) -> ()  [unwired: 1 out]
    n242 = Multiply(x="浓度 2", y=100.0) -> (x*y=w460:dbl)
    n243 = Bundle By Name(cluster=T6 {"starting address"=4224, "number of holding registers"=16}, "starting address"=u16 4224, "number of holding registers"=u16 50) -> (w554:T6)
    n244 = Multiply(x="温度", y=10.0) -> (x*y=w463:dbl)
    n245 = local write "温度 2"(w463) -> ()
    n246 = Multiply(x="修正系数 2", y=100.0) -> (x*y=w457:dbl)
    n247 = local read "Registers"() -> (w548:u16[])
    n248 = Enqueue Element(queue=w496, element=w554, error in (no error)=w495) -> ()  [unwired: 1 in, 3 out]
    n249 = local write "浓度"(w460) -> ()
    n250 = Index Array(array=w548, index #1=0 ("索引"), index #4=3 ("索引"), index #14=13 ("索引"), index #15=14 ("索引"), index #32=31 ("索引")) -> (element #1=w454:u16, element #2=w453:u16, element #3=w452:u16, element #4=w518:u16, element #5=→"模式（受控）":u16, element #6=→"进样管":u16, element #7=→"高锰酸钾":u16, element #8=→"草酸钠":u16, element #9=→"硫酸":u16, element #10=→"ORP显示":u16, element #11=w525:u16, element #12=w527:u16, element #13=w540:u16, element #14=w544:u16, element #15=w498:u16, element #16=w451:u16, element #33=→"分":u16, element #34=→"秒":u16)  [unwired: 29 in, 16 out]
    "多列列表框" <- w451
    n251 = local write "修正系数"(w457) -> ()
    n252 = Divide(x=w544, y=u16 1000) -> (x/y=→"零点滴定值":dbl)
    n253 = Divide(x=w498, y=u16 1000) -> (x/y=→"标度滴定值":dbl)
    n254 = global write "运行时序全局变量.vi" "多列列表框"(w451) -> ()
    n255 = feedback #1(w451) -> (w470:u16)
    n256 = feedback-in #1(w451) -> ()
    n257 = Build Array(w454, w453, w452) -> (w455:u16[])
    n258 = Equal?(x=w527, y=u16 1) -> (x = y?=→"排液标记":bool)
    n259 = Equal?(x=w518, y=u16 0) -> (x = y?=→"待机":bool)
    n260 = Equal?(x=w518, y=u16 7) -> (x = y?=→"质控样测量":bool)
    n261 = Equal?(x=w518, y=u16 1) -> (x = y?=→"水样测量":bool)
    n262 = Equal?(x=w451, y=u16 5) -> (x = y?=w494:bool)
    n263 = Equal?(x=w518, y=u16 9) -> (x = y?=→"校标标记":bool)
    n264 = Equal?(x=w518, y=u16 6) -> (x = y?=→"平行样测量":bool)
    n265 = Equal?(x=w518, y=u16 2) -> (x = y?=→"标样核查标记":bool)
    n266 = Equal?(x=w518, y=u16 8) -> (x = y?=→"校零标记":bool)
    n267 = Equal?(x=w540, y=u16 1) -> (x = y?=w487:bool)
    "ORP故障" <- w487
    n268 = Equal?(x=w540, y=u16 2) -> (x = y?=w486:bool)
    "温控器故障" <- w486
    n269 = Equal?(x=w540, y=u16 3) -> (x = y?=w485:bool)
    "加热故障" <- w485
    n270 = Equal?(x=w540, y=u16 4) -> (x = y?=w484:bool)
    "高锰酸钾报警" <- w484
    n271 = Equal?(x=w540, y=u16 5) -> (x = y?=w483:bool)
    "草酸钠报警" <- w483
    n272 = Equal?(x=w540, y=u16 6) -> (x = y?=w482:bool)
    "测量错误" <- w482
    n273 = Equal?(x=w540, y=u16 8) -> (x = y?=w481:bool)
    "校零错误" <- w481
    n274 = Equal?(x=w540, y=u16 7) -> (x = y?=w480:bool)
    "校标错误" <- w480
    n275 = Equal?(x=w540, y=u16 9) -> (x = y?=w479:bool)
    "进水样超量程" <- w479
    n276 = Divide(x=w525, y=u16 10) -> (x/y=→"温度":dbl)
    n277 = Equal?(x=w518, y=u16 10) -> (x = y?=→"加标回收测量":bool)
    n278 = Equal?(x=w540, y=u16 10) -> (x = y?=w478:bool)
    "排液故障" <- w478
    n279 = Compound Arithmetic op=OR ("复合运算")(w487, w486, w485, w484, w483, w482, w480, w481, w479, w478) -> (→"故障标记":bool)
    n280 = Not Equal?(x=w451, y=w470) -> (x != y?=w469:bool)
    n281 = call <vilib>:"Boolean Crossing PtByPt.vi"("direction"=enum16{"either", "false-true", "true-false"}."false-true", "input"=w494) -> ("crossing"=w492:bool)  [unwired: 1 in]
    n282 = Bundle By Name(cluster=T3 {"ORP故障"=FALSE, "温控器故障"=FALSE, "加热故障"=FALSE, "高锰酸钾报警"=FALSE, "草酸钠报警"=FALSE, "测量错误"=FALSE, "校零错误"=FALSE, "校标错误"=FALSE, " 进水样超量程"=FALSE, "排液阀故障"=FALSE} ("报警簇"), "ORP故障"=w487, "温控器故障"=w486, "加热故障"=w485, "高锰酸钾报警"=w484, "草酸钠报警"=w483, "测量错误"=w482, "校零错误"=w481, "校标错误"=w480, "进水样超量程"=w479, "排液阀故障"=w478) -> (w471:T3)
    "报警簇" <- w471
    n283 = call "HexToDate.vi"("数组"=w455) -> ("DATE"=w449:timestamp[])  [unwired: 10 in]
    n284 = case shown="真" w492 {
      tunnel: w490 -> [_ w628]
      tunnel: w489 -> [_ w623]
      frame False {
      }
      frame True {
        n285 = Bundle By Name(cluster=T6 {"starting address"=0, "number of holding registers"=0}, "starting address"=u16 4101, "number of holding registers"=u16 10) -> (w627:T6)
        n286 = Enqueue Element(queue=w628, element=w627, error in (no error)=w623) -> ()  [unwired: 1 in, 3 out]
        n287 = local write "枚举"(enum16{"读取数据", "写入数据", "读取写入DATABASE", "读取参数"}."读取写入DATABASE" ("枚举")) -> ()
      }
    }
    n288 = case shown="真" w469 {
      tunnel: w451 -> [_ w606]
      frame False {
      }
      frame True {
        n289 = property on="多列列表框" class="MCListbox (严格)"() -> ("ItemNames"=w600:string[][])  [unwired: 2 in, 2 out]
        n290 = Index Array(array=w600, index (row)=w606) -> (element=w597:string[])  [unwired: 1 in]
        n291 = Index Array(array=w597, index=0 ("索引")) -> (element=w595:string)
        n292 = Array To Spreadsheet String(delimiter (Tab)="-" ("分隔符(Tab)"), array=w597, 3:"" ("格式字符串")) -> ()  [unwired: 1 out]
        n293 = Get Date/Time In Seconds() -> (seconds since 1Jan1904=w604:timestamp)
        n294 = Bundle(cluster="data in", "时间标识"=w604, "参数"="CODMn" ("table输入"), "日志信息"=w595, "流程参数"="" ("table输入")) -> (w601:T2)
        n295 = call "流程日志字段定义.vi"("table输入"="操作日志", "data in"=w601) -> ("table输出"=w609:string, "columns"=w610:string[], "data out"=w611:T10)  [unwired: 7 in]
        n296 = call "插入数据.vi"("data"=w611, "columns"=w610, "database"="database3.mdb", "table"=w609) -> ()  [unwired: 7 in, 1 out]
      }
    }
    n297 = Index Array(array=w449) -> (element=→"仪器时间":timestamp)  [unwired: 1 in]
    n298 = Get Date/Time In Seconds() -> (seconds since 1Jan1904=w448:timestamp)
    "系统时间" <- w448
    n299 = global read "COD读取DATA全局.vi" "data"() -> (w431:T5)
    n300 = global read "COD测量模式全局.vi" "测量模式"() -> (w430:string)
    n301 = Build Array(w448) -> (w447:timestamp[])
    n302 = Unbundle By Name(w431) -> ("时间"=w428:timestamp, "检测值"=w427:sgl, "数据标识"=w426:string)
    n303 = call "DateToHex.vi"("DATE"=w447) -> ("数组"=w446:u16[])  [unwired: 10 in]
    n304 = call "DateToHex.vi"("DATE"=w449) -> ("数组"=w441:u16[])  [unwired: 10 in]
    n305 = local read "测量数据区"() -> (w432:T1)
    n306 = case shown="\"标样核查\"" w430 {
      tunnel: w432 -> [w555 w560 w565 w570 w575 w580 w585 w590]
      tunnel: [w555 w559 w561 w569 w574 w579 w581 w589] -> w429
      tunnel: w428 -> [_ w558 w564 w568 w573 w578 w584 w588]
      tunnel: w427 -> [_ w557 w563 w567 w572 w577 w583 w587]
      tunnel: w426 -> [_ w556 w562 w566 w571 w576 w582 w586]
      frame "", Default {
      }
      frame "水样测试" {
        n307 = Bundle By Name(cluster=w560, "水样数据时间"=w558, "水样实测值"=w557, "水样数据标识"=w556) -> (w559:T1)
      }
      frame "标样核查" {
        n308 = Bundle By Name(cluster=w565, "跨度核查数据时间"=w564, "跨度核查实测值"=w563, "跨度核查数据标识"=w562) -> (w561:T1)
      }
      frame "零点核查" {
        n309 = Bundle By Name(cluster=w570, "零点核查数据时间"=w568, "零点核查实测值"=w567, "零点核查数据标识"=w566) -> (w569:T1)
      }
      frame "加标回收" {
        n310 = Bundle By Name(cluster=w575, "加标回收数据时间"=w573, "加标回收实测值"=w572, "加标回收数据标识"=w571) -> (w574:T1)
      }
      frame "平行样" {
        n311 = Bundle By Name(cluster=w580, "平行样数据时间"=w578, "平行样实测值"=w577, "平行样数据标识"=w576) -> (w579:T1)
      }
      frame "校零" {
        n312 = Bundle By Name(cluster=w585, "空白数据时间"=w584, "空白实测值"=w583, "空白数据标识"=w582) -> (w581:T1)
      }
      frame "校标" {
        n313 = Bundle By Name(cluster=w590, "标样数据时间"=w588, "标样实测值"=w587, "标样数据标识"=w586) -> (w589:T1)
      }
    }
    "测量数据区" <- w429
    n314 = Index Array(array=w441, index=2 ("索引")) -> (element=w443:u16)
    n315 = Index Array(array=w446, index=2 ("索引")) -> (element=w444:u16)
    n316 = Split Number(x=w443) -> (hi(x)=w437:u8)  [unwired: 1 out]
    n317 = call "CODMn报警信息.vi"("报警簇"=w471) -> ("CODMN报警信息"=w472:string)  [unwired: 10 in]
    n318 = Split Number(x=w444) -> (hi(x)=w440:u8)  [unwired: 1 out]
    n319 = To Byte Integer(number=w437) -> (8bit integer=w436:i8)
    n320 = To Byte Integer(number=w440) -> (8bit integer=w439:i8)
    n321 = Subtract(x=w436, y=w439) -> (x-y=w438:i8)
    n322 = feedback #2(w472) -> (w473:string)
    n323 = feedback-in #2(w472) -> ()
    n324 = Not Equal?(x=w472, y="") -> (x != y?=w477:bool)
    n325 = Absolute Value(x=w438) -> (abs(x)=w435:i8)
    n326 = Greater Or Equal?(x=w435, y=i8 5) -> (x >= y?=w433:bool)
    n327 = Not Equal?(x=w472, y=w473) -> (x != y?=w474:bool)
    n328 = case shown="真" w433 {
      tunnel: w433 -> [_ w591]
      frame False {
      }
      frame True {
        n329 = flat-sequence {
          tunnel: w591 -> [_]
          frame #0 {
            n330 = property on="时间校准" class="Bool (严格)"("Val(Sgnl)"=TRUE ("时间校准")) -> ()  [unwired: 2 in, 2 out]
          }
          frame #1 {
            n331 = Wait (ms)(milliseconds to wait=u32 300 ("等待时间（毫秒）")) -> ()  [unwired: 1 out]
          }
          frame #2 {
            n332 = property on="时间校准" class="Bool (严格)"("Val(Sgnl)"=FALSE ("时间校准")) -> ()  [unwired: 2 in, 2 out]
          }
        }
      }
    }
    n333 = And(x=w474, y=w477) -> (x .and. y?=w475:bool)
    n334 = case shown="真" w475 {
      tunnel: w472 -> [_ w612]
      frame False {
      }
      frame True {
        n335 = Get Date/Time In Seconds() -> (seconds since 1Jan1904=w614:timestamp)
        n336 = Bundle By Name(cluster=T9 {"时间标识"=timestamp(0 s since 1904-01-01), "设备"="", "日志信息"=""} ("data in"), "时间标识"=w614, "设备"="CODMn", "日志信息"=w612) -> (w615:T9)
        n337 = call "报警信息字段定义.vi"("table输入"="报警信息", "data in"=w615) -> ("table输出"=w619:string, "columns"=w620:string[], "data out"=w621:T9)  [unwired: 7 in]
        n338 = call "插入数据.vi"("data"=w621, "columns"=w620, "database"="database3.mdb", "table"=w619) -> ()  [unwired: 7 in, 1 out]
      }
    }
    "循环次数" <- w491
  }
  n339 = call-dynamic "Close Session.vi"("error in (no error)"=w18, "MB_Serial session"=w17) -> ()  [unwired: 9 in, 1 out]
